vi "JSON Object.vi"(8 "error in (no error)":errorcluster, 10 "Start Index":i32, 11 "JSON":string) -> (0 "error out":errorcluster, 2 "End Index":i32, 3 "VCluster":variant)   [LabVIEW 2011]
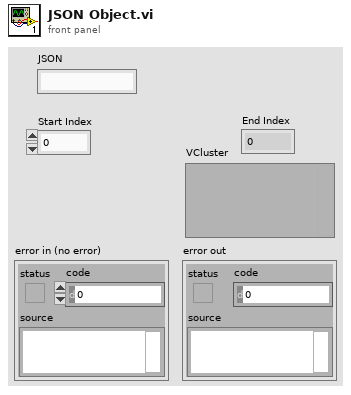
[diagram p1: front panel]
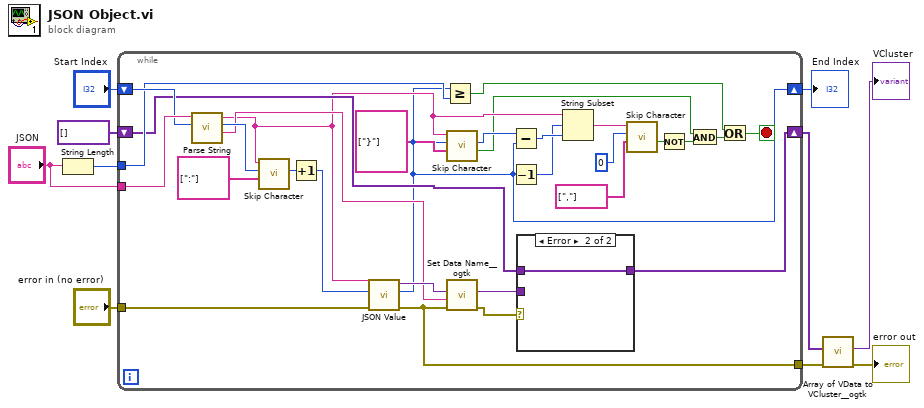
[diagram p0: block diagram]
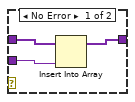
[diagram p2: hidden frame]
diagram:
  n1 = String Length(string="JSON") -> (length=w7:i32)
  n2 = while {
    tunnel: "JSON" -> [w40]
    shift-right: [w20] -> w9
    shift-left: "Start Index" -> [w39]
    tunnel: w7 -> [w32]
    shift-right: [w27] -> w5
    shift-left: variant[] [] -> [w28]
    tunnel: "error in (no error)" -> [w13]
    tunnel: [w11] -> w2
    stop <- w14 stop-if-true
    n3 = call "Parse String.vi"("Start Index"=w39, "JSON"=w40) -> ("String"=w29:string, "EndIndex"=w38:i32, "JSON"=w25:string)  [unwired: 6 in]
    n4 = call "Skip Character.vi"("Stop Strings"=string[] [":"], "Start Index"=w38, "JSON"=w25) -> ("End Index"=w36:u32)  [unwired: 6 in, 2 out]
    n5 = Increment(x=w36) -> (x+1=w35:u32)
    n6 = call "JSON Value.vi"("error in (no error)"=w13, "Start Index"=w35, "JSON"=w25) -> ("error out"=w11:errorcluster, "End Index"=w20:u32, "Value"=w30:variant)  [unwired: 6 in]
    n7 = Greater Or Equal?(x=w20, y=w32) -> (x >= y?=w33:bool)
    n8 = call "Skip Character.vi"("Stop Strings"=string[] ["}"], "Start Index"=w20, "JSON"=w25) -> ("Found Stop Character"=w19:bool, "End Index"=w24:u32)  [unwired: 6 in, 1 out]
    n9 = call <userlib>:"Set Data Name__ogtk.vi"("error in (no error)"=w11, "Data Name"=w29, "Data"=w30) -> ("error out"=w12:errorcluster, "Renamed Data"=w26:variant)  [unwired: 7 in]
    n10 = Subtract(x=w24, y=w20) -> (x-y=w23:u32)
    n11 = Decrement(x=w20) -> (x-1=w16:u32)
    n12 = case shown="Error" w12 {
      tunnel: w28 -> [w43 w44]
      tunnel: [w42 w44] -> w27
      tunnel: w26 -> [w41 _]
      frame No Error {
        n13 = Insert Into Array(array=w43, new element=w41) -> (w42:variant[])  [unwired: 1 in]
      }
      frame Error {
      }
    }
    n14 = String Subset(string=w25, offset (0)=w16, length (rest)=w23) -> (substring=w22:string)
    n15 = call "Skip Character.vi"("Stop Strings"=string[] [","], "Start Index"=u32 0, "JSON"=w22) -> ("Found Stop Character"=w18:bool)  [unwired: 6 in, 2 out]
    n16 = Not(x=w18) -> (.not. x?=w17:bool)
    n17 = And(x=w19, y=w17) -> (x .and. y?=w31:bool)
    n18 = Or(x=w33, y=w31) -> (x .or. y?=w14:bool)
  }
  "End Index" <- w9
  n19 = call <userlib>:"Array of VData to VCluster__ogtk.vi"("error in (no error)"=w2, "Array"=w5) -> ("error out"=→"error out":errorcluster, "VCluster"=→"VCluster":variant)  [unwired: 8 in]
